vi "Create Test File And Compile It.vi"(8 "Error In":errorcluster, 9 "text":string="#include <stdio.h>\n#include \"example_dll.h\"\n\nint main(void)\n{\n        //LuboJ. don't forget LabVIEW transcriptor prefix for SubVIs!\n        \n        LVSubVI_CppFunc();                            //there is used in call generated function prefix LVSubVI_\n        for(int i = 0; i < 200; i++){\n                //there is used in call generated function prefix LVSubVI_\n                printf(\"%d\\n\", LVSubVI_Double(i));\n        }\n\n        return 0;\n}\n", 10 "MinGW Path":path=path "C:/Program Files/mingw-w64/x86_64-8.1.0-posix-seh-rt_v6-rev0/mingw64/bin", 11 "generated DLL lib path":path) -> (0 "Error Out":errorcluster, 2 "standard error":string, 3 "standard output":string)   [LabVIEW 2014]
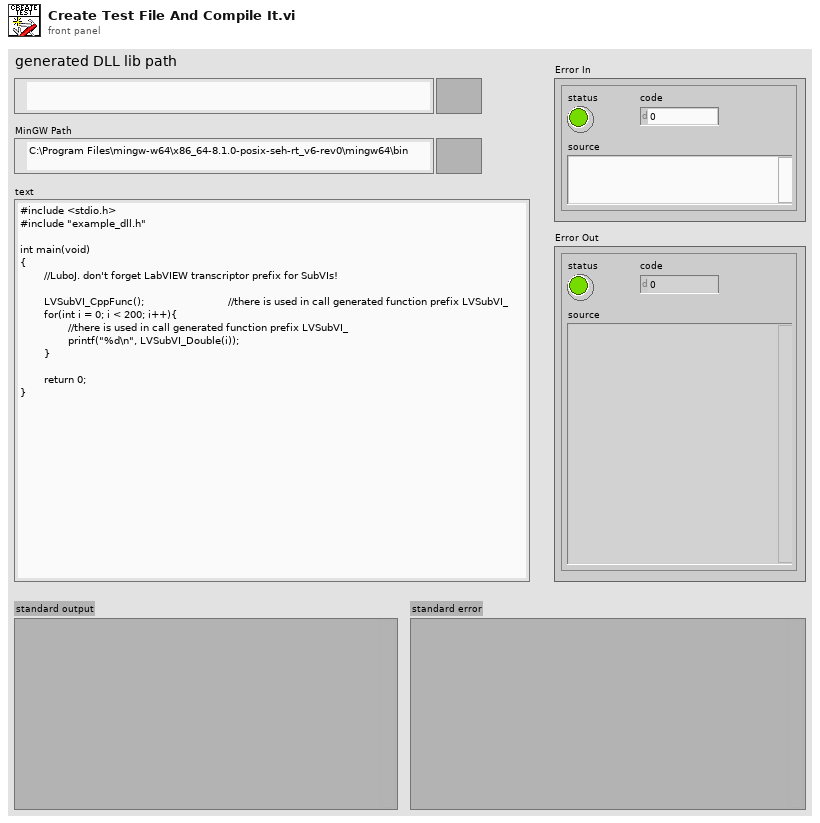
[diagram p1: front panel]
types:
  T1 = enum16{"open", "replace", "create", "open or create", "replace or create", "replace or create with confirmation"}
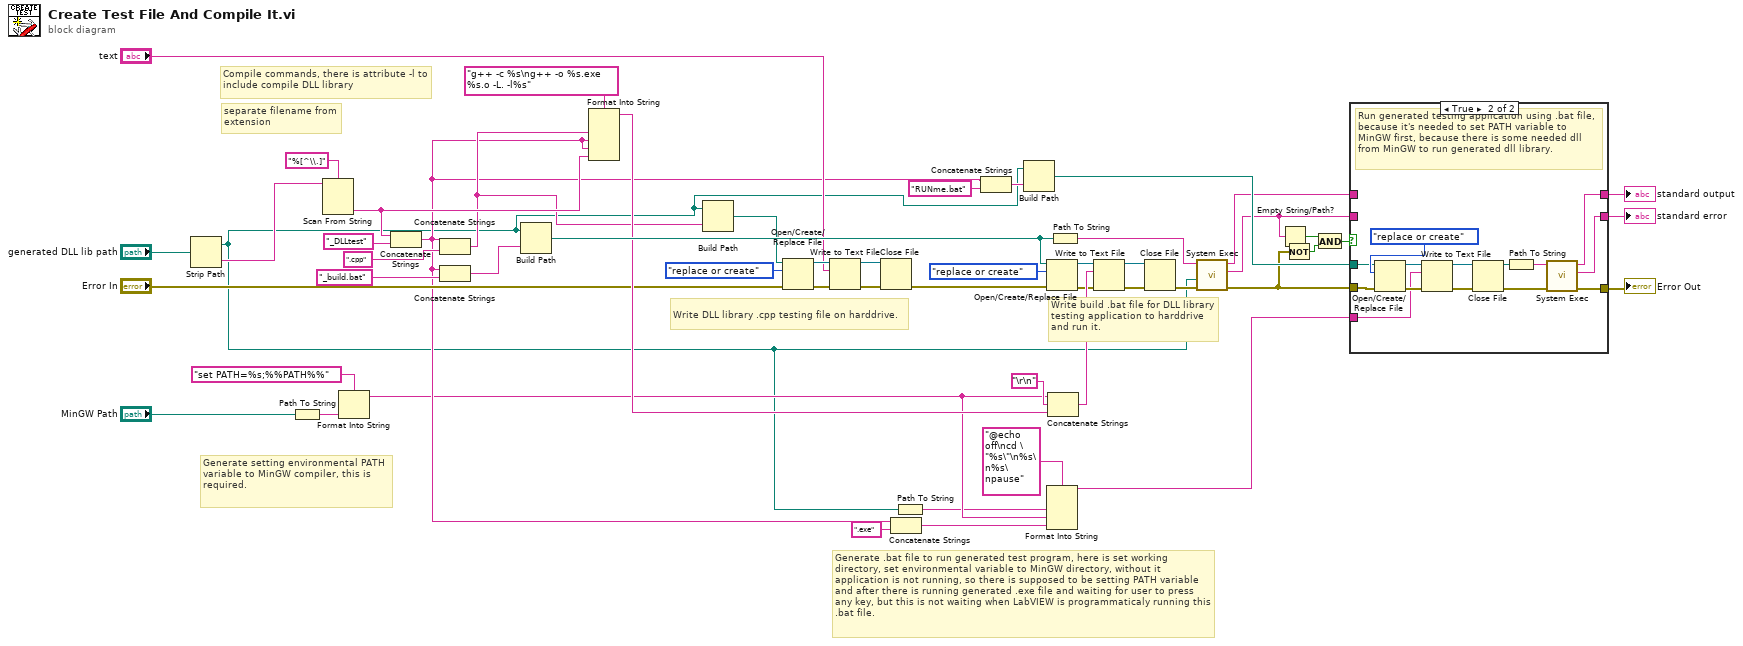
[diagram p0: block diagram]
diagram:
  # "Write build .bat file for DLL library testing application to harddrive and run it."
  # "Write DLL library .cpp testing file on harddrive."
  # "separate filename from extension"
  # "Compile commands, there is attribute -l to include compile DLL library"
  # "Generate setting environmental PATH variable to MinGW compiler, this is required."
  # "Generate .bat file to run generated test program, here is set working directory, set environmental variable to MinGW directory, without it application is not running, so there is supposed to be setting PATH variable and after there is running generated .exe file and waiting for user to press any key, but this is not waiting when LabVIEW is programmaticaly running this .bat file."
  n1 = Strip Path(path="generated DLL lib path") -> (stripped path=w6:path, name=w38:string)
  n2 = Path To String(path="MinGW Path") -> (string=w51:string)
  n3 = Scan From String(format string="%[^\\.]", input string=w38) -> (output 1=w35:string)  [unwired: 3 in, 3 out]
  n4 = Format Into String(format string="set PATH=%s;%%PATH%%" ("command line"), w51) -> (resulting string=w8:string)  [unwired: 2 in, 1 out]
  n5 = Concatenate Strings(w35, "_DLLtest" ("string")) -> (w17:string)
  n6 = Concatenate Strings(w17, ".cpp" ("string")) -> (w23:string)
  n7 = Concatenate Strings(w17, "_build.bat" ("string")) -> (w31:string)
  n8 = Build Path(base path=w6, name or relative path=w31) -> (appended path=w41:path)
  n9 = Format Into String(format string="g++ -c %s\ng++ -o %s.exe %s.o -L. -l%s" ("string"), w23, w17, w17, w35) -> (resulting string=w34:string)  [unwired: 2 in, 1 out]
  n10 = Build Path(base path=w6, name or relative path=w23) -> (appended path=w22:path)
  n11 = Open/Create/Replace File(file path (use dialog)=w22, error in="Error In", operation (0:open)=T1."replace or create") -> (refnum out=w28:refnum<file>, error out=w27:errorcluster)  [unwired: 3 in, 1 out]
  n12 = Write to Text File(file (use dialog)=w28, text="text", error in=w27) -> (refnum out=w30:refnum<file>, error out=w29:errorcluster)  [unwired: 1 in, 1 out]
  n13 = Close File(refnum=w30, error in=w29) -> (error out=w25:errorcluster)  [unwired: 1 out]
  n14 = Concatenate Strings(w17, ".exe" ("string")) -> (w9:string)
  n15 = Path To String(path=w6) -> (string=w7:string)
  n16 = Concatenate Strings(w17, "RUNme.bat" ("string")) -> (w19:string)
  n17 = Build Path(base path=w6, name or relative path=w19) -> (appended path=w18:path)
  n18 = Open/Create/Replace File(file path (use dialog)=w41, error in=w25, operation (0:open)=T1."replace or create") -> (refnum out=w46:refnum<file>, error out=w47:errorcluster)  [unwired: 3 in, 1 out]
  n19 = Format Into String(format string="@echo off\ncd \"%s\"\n%s\n%s\npause", w7, w8, w9) -> (resulting string=w13:string)  [unwired: 2 in, 1 out]
  n20 = Concatenate Strings(w8, "\r\n", w34) -> (w48:string)
  n21 = Path To String(path=w41) -> (string=w40:string)
  n22 = Write to Text File(file (use dialog)=w46, text=w48, error in=w47) -> (refnum out=w44:refnum<file>, error out=w45:errorcluster)  [unwired: 1 in, 1 out]
  n23 = Close File(refnum=w44, error in=w45) -> (error out=w42:errorcluster)  [unwired: 1 out]
  n24 = call <vilib>:"System Exec.vi"("error in (no error)"=w42, "working directory"=w6, "command line"=w40) -> ("error out"=w1:errorcluster, "standard error"=w3:string, "standard output"=w10:string)  [unwired: 5 in, 1 out]
  n25 = Empty String/Path?(string/path=w3) -> (empty?=w4:bool)
  n26 = Not(x=w1) -> (.not. x?=w2:bool)
  n27 = And(x=w4, y=w2) -> (x .and. y?=w5:bool)
  n28 = case shown="True" w5 {
    tunnel: w18 -> [_ w65]
    tunnel: [w54 w63] -> w15
    tunnel: w13 -> [_ w64]
    tunnel: [w56 w59] -> w12
    tunnel: w3 -> [w56 _]
    tunnel: [w55 w58] -> w11
    tunnel: w10 -> [w55 _]
    tunnel: w1 -> [w54 w57]
    frame False {
    }
    frame True {
      # "Run generated testing application using .bat file, because it's needed to set PATH variable to MinGW first, because there is some needed dll from MinGW to run generated dll library."
      n29 = Open/Create/Replace File(file path (use dialog)=w65, error in=w57, operation (0:open)=T1."replace or create") -> (refnum out=w68:refnum<file>, error out=w67:errorcluster)  [unwired: 3 in, 1 out]
      n30 = Write to Text File(file (use dialog)=w68, text=w64, error in=w67) -> (refnum out=w70:refnum<file>, error out=w69:errorcluster)  [unwired: 1 in, 1 out]
      n31 = Close File(refnum=w70, error in=w69) -> (path=w61:path, error out=w62:errorcluster)
      n32 = Path To String(path=w61) -> (string=w60:string)
      n33 = call <vilib>:"System Exec.vi"("error in (no error)"=w62, "command line"=w60) -> ("error out"=w63:errorcluster, "standard error"=w59:string, "standard output"=w58:string)  [unwired: 6 in, 1 out]
    }
  }
  "Error Out" <- w15
  "standard output" <- w11
  "standard error" <- w12
